vi "GE 5565PIORC.Open.vi"() -> (0 "error out":errorcluster, 3 "GE 5565PIORC":refnum<class "GE 5565PIORC.lvclass">)   [LabVIEW 2020]
uses:
  Source/GE 5565PIORC.lvclass
  Source/GE 5565PIORC.lvclass/GE 5565PIORC.ctl
  Source/Properties/Registers/GE 5565PIORC.Registers.LAS1RR.PCI Address Range.Get.vi
  Source/Methods/GE 5565PIORC.PXI Interrupts.Enable.vi
  Source/Properties/Registers/GE 5565PIORC.Registers.Local Configuration.Read.vi
  Source/Properties/Registers/GE 5565PIORC.Registers.Local Configuration.Read (U32).vi
  Source/Methods/GE 5565PIORC.Registers.Read.vi
  Source/Methods/GE 5565PIORC.Registers.Read (U32).vi
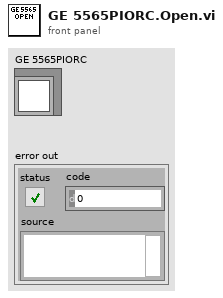
[diagram p1: front panel]
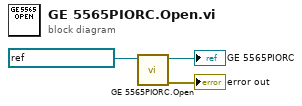
[diagram p0: block diagram]
diagram:
  n1 = call "GE 5565PIORC.Open.vi"("VISA resource name"=refnum<visa-resource-name> "PXI4::14::INSTR") -> ("error out"=→"error out":errorcluster, "GE 5565PIORC"=→"GE 5565PIORC":refnum<class "GE 5565PIORC.lvclass">)  [unwired: 9 in]
